vi "theta_upd.vi"(0 "\\phi(t)":T1, 1 "P(t)":T1, 2 "\\eps_0(t)":dbl, 3 "\\theta(t-1)":T1, 4 "error in (no error)":errorcluster) -> (5 "\\theta(t)":T1, 6 "error out":errorcluster)   [LabVIEW 2021]
uses:
  <vilib>/Analysis/Matrix/Datatypes/RealMatrix.ctl
  <vilib>/Analysis/Matrix/Numeric/Multiply/Multiply - RM,RM.vi
  <vilib>/Analysis/Matrix/Numeric/Multiply/Multiply - RM,R.vi
  <vilib>/Analysis/Matrix/Numeric/Add/Add - RM,RM.vi
  <vilib>/Analysis/Matrix/NI_Matrix.lvlib
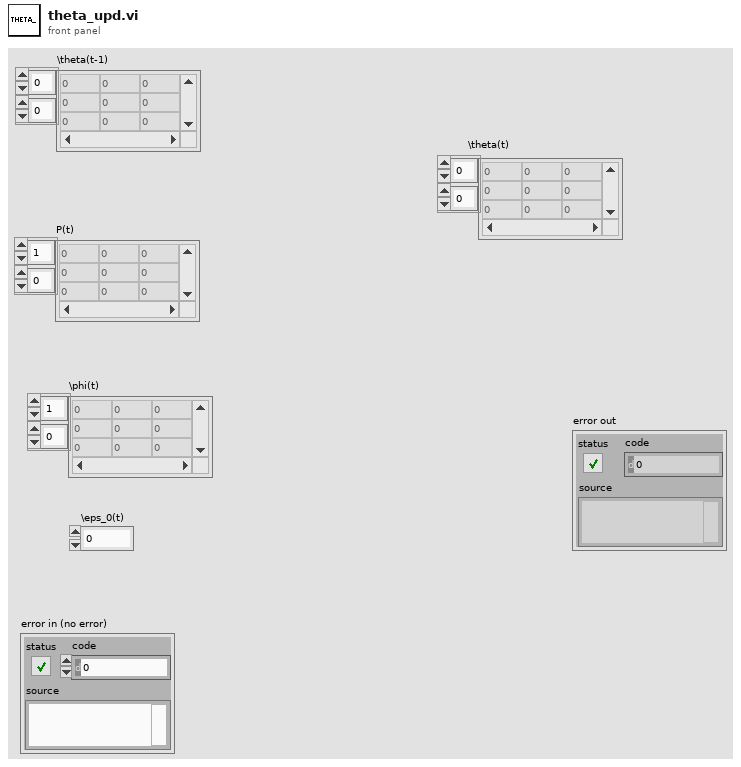
[diagram p1: front panel]
types:
  T1 = typedef "NI_Matrix.lvlib/RealMatrix.ctl" = dbl[][]
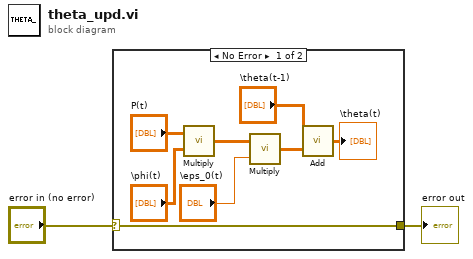
[diagram p0: block diagram]
diagram:
  n1 = case shown="No Error" "error in (no error)" {
    selector: "error in (no error)" -> [w3 w11]
    tunnel: [w3 w11] -> w1
    frame No Error {
      n2 = call-poly <vilib>:"Multiply.vi"("Real Matrix B"="\\phi(t)", "Real Matrix A"="P(t)") -> ("A * B"=w7:T1)
      n3 = call-poly <vilib>:"Multiply.vi"("Real Scalar c"="\\eps_0(t)", "Real Matrix A"=w7) -> ("A * c"=w5:T1)
      n4 = call-poly <vilib>:"Add.vi"("Real Matrix B"=w5, "Real Matrix A"="\\theta(t-1)") -> ("A + B"=→"\\theta(t)":T1)
    }
    frame Error {
    }
  }
  "error out" <- w1
